vi "PressureCal.vi"(8 "Motion Settings In":T5={"No Motion?"=FALSE, "Motion System"=enum."No Motion Card", "Motion Bd ID"=1, "Motion Profile"="SMAC1", "# Axis"=1, "Reverse Z axis?"=TRUE, "SMAC Axis"=0, "scan pair"=enum."y-(x) scan", "RT fps"=6.0, "Steps per mm"=[1000, 1000, 1000, 1000], "Motor Parameters"={"velocity ct/s"=[10000.0, 10000.0, 10000.0, 50000.0], "accel ct/s^2"=[50000.0, 50000.0, 50000.0, 200000.0]}, "One Way Scan"=FALSE, "Reverse One Way Scan"=FALSE, "Global Position (mm)"=[], "Plane"=0, "Distance between\nscan lines (um)"=0.0, "Distance between\nscan planes (um)"=0.0, "number of scan planes"=1, "Total steps in line"=0, "Xtra plane\ndistance  (um)"=100, "Xtra planes "=1, "Add Axis"=FALSE, "overshoot cts"=200, "BKPT Shift"=0, "Scan Start Time (ms)"=0, "ESP VISA"="GPIB::1::INSTR", "3rd Axis"=1, "GL Ref Out"=refnum, "Galil Address"=""} {"3rd Axis" items=["x", "y", "z", "w"]; "Xtra planes" min=1; "Xtra plane\ndistance  (um)" min=0; "Distance between\nscan planes (um)" format="%.2f"; "Distance between\nscan lines (um)" format="%.2f"; "SMAC Axis" items=["None"=0, "Axis 1"=1, "Axis 2"=2, "Axis 3"=3, "Axis 4"=4, "Axis 5"=5, "Axis 6"=6, "Axis 7"=7, "Axis 8"=8, "Vector Space 1"=17, "Vector Space 2"=18, "Vector Space 3"=19, "Vector Space 4"=20]; "Motion Bd ID" min=1 max=32 step=1}, 9 "Burst Select":bool=TRUE, 10 "FG Source":u16(ring)=1 items=["Agilent"=2, "Tabor"=7, ""=0], 11 "Digitizer Settings":T1={"Digitizer delay (us) "=0.0, "rf points per line"=2048, "lines per plane"=128, "Samp Rate (Hz)"=100000000.0, "Additional dig delay (us)"=0.0, "Voltage Scale"=0.4, "Pre-Looks"=0, "Offset delay (us)"=0.0, "bits A/D"=8, "Avg Num"=1, "DigTimeOut"=5.0, "Rel Dig Delay"=0.0, "Dig Ch"=0, "LeCroyCluster"={"LeCroy Channels"=[TRUE, FALSE, FALSE, FALSE], "LC read pt offset"=0.0, "Sweep Avg"=FALSE}, "Main Digitizer"=enum."NI Digitizer", "Dig Config"=enum."Single channel", "Digitizer ID Cluster"={"Acqiris/Alazar/SP ID"=[], "NI Instr Handles"=[], "LeCroy VISA"="", "GaGe Handle"={"Handle"=0, "Sample size"=0, "Resolution"=0, "Offset"=0, "Channels"=0, "Boards"=0}, "ATS Ref"="ATS9350", "Acqiris Address"=["PCI::INSTR0"], "ADQRef"=refnum, "adq_cu_ptr"=refnum}, "Trigger Settings"={"Trig Source"=1, "Trig Coupling"=0, "Trig Slope"=0, "Level (mV)"=1500.0}, "Bulk Acq"=FALSE, "Bulk Start Indexes"=[], "Data Ref RF"=refnum, "NI ID/Channel"=[], "Total Dig CH"=5, "Xtra Ann Trig delay (us)"=10.0, "Fix Z Delay?"=FALSE, "One Way Transmission?"=FALSE, "Data Ref Log"=refnum} {"Trigger Settings"."Trig Slope" items=["Positive", "Negative"]; "Trigger Settings"."Level (mV)" format="%.2f"; "Trigger Settings"."Trig Coupling" items=["DC 1 MOhm", "AC 1 MOhm", "DC 50 Ohm", "AC 50 Ohm"]; "Trigger Settings"."Trig Source" items=["Chan 1", "External"]; "Rel Dig Delay" format="%.2f"; "DigTimeOut" format="%.2f"; "Avg Num" min=1; "Offset delay (us)" format="%.2f"; "Additional dig delay (us)" format="%.2f"; "Digitizer delay (us)" format="%.2f"}) -> (0 "Motion Settings Out":T5={"No Motion?"=FALSE, "Motion System"=enum."No Motion Card", "Motion Bd ID"=1, "Motion Profile"="SMAC1", "# Axis"=1, "Reverse Z axis?"=TRUE, "SMAC Axis"=0, "scan pair"=enum."y-(x) scan", "RT fps"=6.0, "Steps per mm"=[1000, 1000, 1000, 1000], "Motor Parameters"={"velocity ct/s"=[10000.0, 10000.0, 10000.0, 50000.0], "accel ct/s^2"=[50000.0, 50000.0, 50000.0, 200000.0]}, "One Way Scan"=FALSE, "Reverse One Way Scan"=FALSE, "Global Position (mm)"=[], "Plane"=0, "Distance between\nscan lines (um)"=0.0, "Distance between\nscan planes (um)"=0.0, "number of scan planes"=1, "Total steps in line"=0, "Xtra plane\ndistance  (um)"=100, "Xtra planes "=1, "Add Axis"=FALSE, "overshoot cts"=200, "BKPT Shift"=0, "Scan Start Time (ms)"=0, "ESP VISA"="GPIB::1::INSTR", "3rd Axis"=1, "GL Ref Out"=refnum, "Galil Address"=""} {"3rd Axis" items=["x", "y", "z", "w"]; "Xtra planes" min=1; "Xtra plane\ndistance  (um)" min=0; "Distance between\nscan planes (um)" format="%.2f"; "Distance between\nscan lines (um)" format="%.2f"; "SMAC Axis" items=["None"=0, "Axis 1"=1, "Axis 2"=2, "Axis 3"=3, "Axis 4"=4, "Axis 5"=5, "Axis 6"=6, "Axis 7"=7, "Axis 8"=8, "Vector Space 1"=17, "Vector Space 2"=18, "Vector Space 3"=19, "Vector Space 4"=20]; "Motion Bd ID" min=1 max=32 step=1}, 3 "Digitizer Settings Out":T1={"Digitizer delay (us) "=0.0, "rf points per line"=2048, "lines per plane"=128, "Samp Rate (Hz)"=100000000.0, "Additional dig delay (us)"=0.0, "Voltage Scale"=0.4, "Pre-Looks"=0, "Offset delay (us)"=0.0, "bits A/D"=8, "Avg Num"=1, "DigTimeOut"=5.0, "Rel Dig Delay"=0.0, "Dig Ch"=0, "LeCroyCluster"={"LeCroy Channels"=[TRUE, FALSE, FALSE, FALSE], "LC read pt offset"=0.0, "Sweep Avg"=FALSE}, "Main Digitizer"=enum."NI Digitizer", "Dig Config"=enum."Single channel", "Digitizer ID Cluster"={"Acqiris/Alazar/SP ID"=[], "NI Instr Handles"=[], "LeCroy VISA"="", "GaGe Handle"={"Handle"=0, "Sample size"=0, "Resolution"=0, "Offset"=0, "Channels"=0, "Boards"=0}, "ATS Ref"="ATS9350", "Acqiris Address"=["PCI::INSTR0"], "ADQRef"=refnum, "adq_cu_ptr"=refnum}, "Trigger Settings"={"Trig Source"=1, "Trig Coupling"=0, "Trig Slope"=0, "Level (mV)"=1500.0}, "Bulk Acq"=FALSE, "Bulk Start Indexes"=[], "Data Ref RF"=refnum, "NI ID/Channel"=[], "Total Dig CH"=5, "Xtra Ann Trig delay (us)"=10.0, "Fix Z Delay?"=FALSE, "One Way Transmission?"=FALSE, "Data Ref Log"=refnum} {"Trigger Settings"."Trig Slope" items=["Positive", "Negative"]; "Trigger Settings"."Level (mV)" format="%.2f"; "Trigger Settings"."Trig Coupling" items=["DC 1 MOhm", "AC 1 MOhm", "DC 50 Ohm", "AC 50 Ohm"]; "Trigger Settings"."Trig Source" items=["Chan 1", "External"]; "Rel Dig Delay" format="%.2f"; "DigTimeOut" format="%.2f"; "Avg Num" min=1; "Offset delay (us)" format="%.2f"; "Additional dig delay (us)" format="%.2f"; "Digitizer delay (us)" format="%.2f"})   [LabVIEW 2022 SP3]
uses:
  -CalTransducer/HydrophoneSettings.ctl
  -CalTransducer/Hydros.ctl
  ScanningControl/Digitizers/-DigitizerRoutines/DigitizerSettings.ctl
  ScanningControl/Digitizers/-DigitizerRoutines/Digitizer.ctl
  ScanningControl/Digitizers/-DigitizerRoutines/DigConfig.ctl
  ScanningControl/Digitizers/-DigitizerRoutines/DigitizerID.ctl
  C:/Windows/System32/ADQAPI_dotNet_helper.dll
  ScanningControl/Motion Controllers/NI_controller/-NI_MotionRoutines/MotionParameters.ctl
  ScanningControl/Motion Controllers/NI_controller/-NI_MotionRoutines/MotionSys.ctl
  ScanningControl/Motion Controllers/-MotionRoutines/ScanAxis.ctl
  ScanningControl/Motion Controllers/-MotionRoutines/3rdAxis.ctl
  ScanningControl/-ScanSystem/Controls/ScanType2.ctl
  <vilib>/DAQmx/write.llb/DAQmx Write (Digital 1D Bool NChan 1Samp 1Line).vi
  <vilib>/Analysis/5stat.llb/RMS (DBL).vi
  <vilib>/Analysis/baseanly.llb/Mean (DBL).vi
  <vilib>/DAQmx/miscellaneous.llb/DAQmx Fill In Error Info.vi
  <instrlib>/niScope/Acquire/Fetch/niScope Fetch.vi
  <vilib>/Utility/file.llb/Write Delimited Spreadsheet (DBL).vi
  <instrlib>/Acqiris Dx/Acqiris Dx.lvlib
  <vilib>/Analysis/NI_AALPro.lvlib
  <vilib>/Analysis/NI_AALBase.lvlib
panel:
  in  "Invert PAL voltage":bool=TRUE
  out "f (MHz)":dbl
  in  "Freq Step to View":u8
  in  "V probe":u16(ring)=1 items=["1x"=1, "10x"=10, "100x"=100]
  in  "Start freq (MHz)":dbl=1.0 format="%.2f"
  in  "Freq Steps":u32=1
  in  "Average":i32=1
  in  "Freq Step (MHz":dbl=2.0 format="%.2f"
  in  "Cal Tran":bool
  in  "Set up Digi":bool
  in  "ExitSendCmd":bool
  in  "Save Cal Data":bool
  in  "Save RF array?":bool
  in  "Pressure Cal Parameters":T9={"Center Freq (MHz)"=40.0, "PRF (kHz)"=1.0, "Pulse window (us)"=0.5, "Hydrophone"=enum."DEAD PAL # 1403", "booster amp?"=TRUE} {"Pulse window (us)" format="%.2f"; "PRF (kHz)" format="%.2f"; "Center Freq (MHz)" format="%.2f"}
  in  "Voltage Step (mVpp)":dbl=10.0 format="%.2f"
  in  "Voltage Steps":i32=20
  in  "Start voltage (mVpp)":dbl=50.0 format="%.3f"
  out "RMS dB ratio":cluster{"V Steps":dbl[], "RMS Ratio":dbl[]}(graph)
  out "current f (MHz)":dbl
  out "Voltage + pk and -pk":dbl[][](graph)
  out "Raw RF":dbl[][](array[numeric])
  out "Cal Array":dbl[][](array[numeric])
  out "Mpa/V":dbl format="%.2f"
  out "Voltage at Transducer":cluster{dbl[], dbl[]}(graph)
  out "Hydrophone":cluster{"V Steps":dbl[], dbl[]}[](graph)
  out "slope":dbl format="%.2f"
  out "intercept":dbl format="%.2f"
  out "mse":dbl format="%.2f"
  out "current Vpp":dbl
  # "***Voltages are inverted for PAL 40 um hydrophones***"
  # ")"
  # "Fit Params for hydrophone"
  # "FG drive\nvoltage matching (Vpp)\nvolt hydrop V\nPressure  neg MPa"
  # "1-D and 2-D B scan settings"
  # "1-D and 2-D B scan settings"
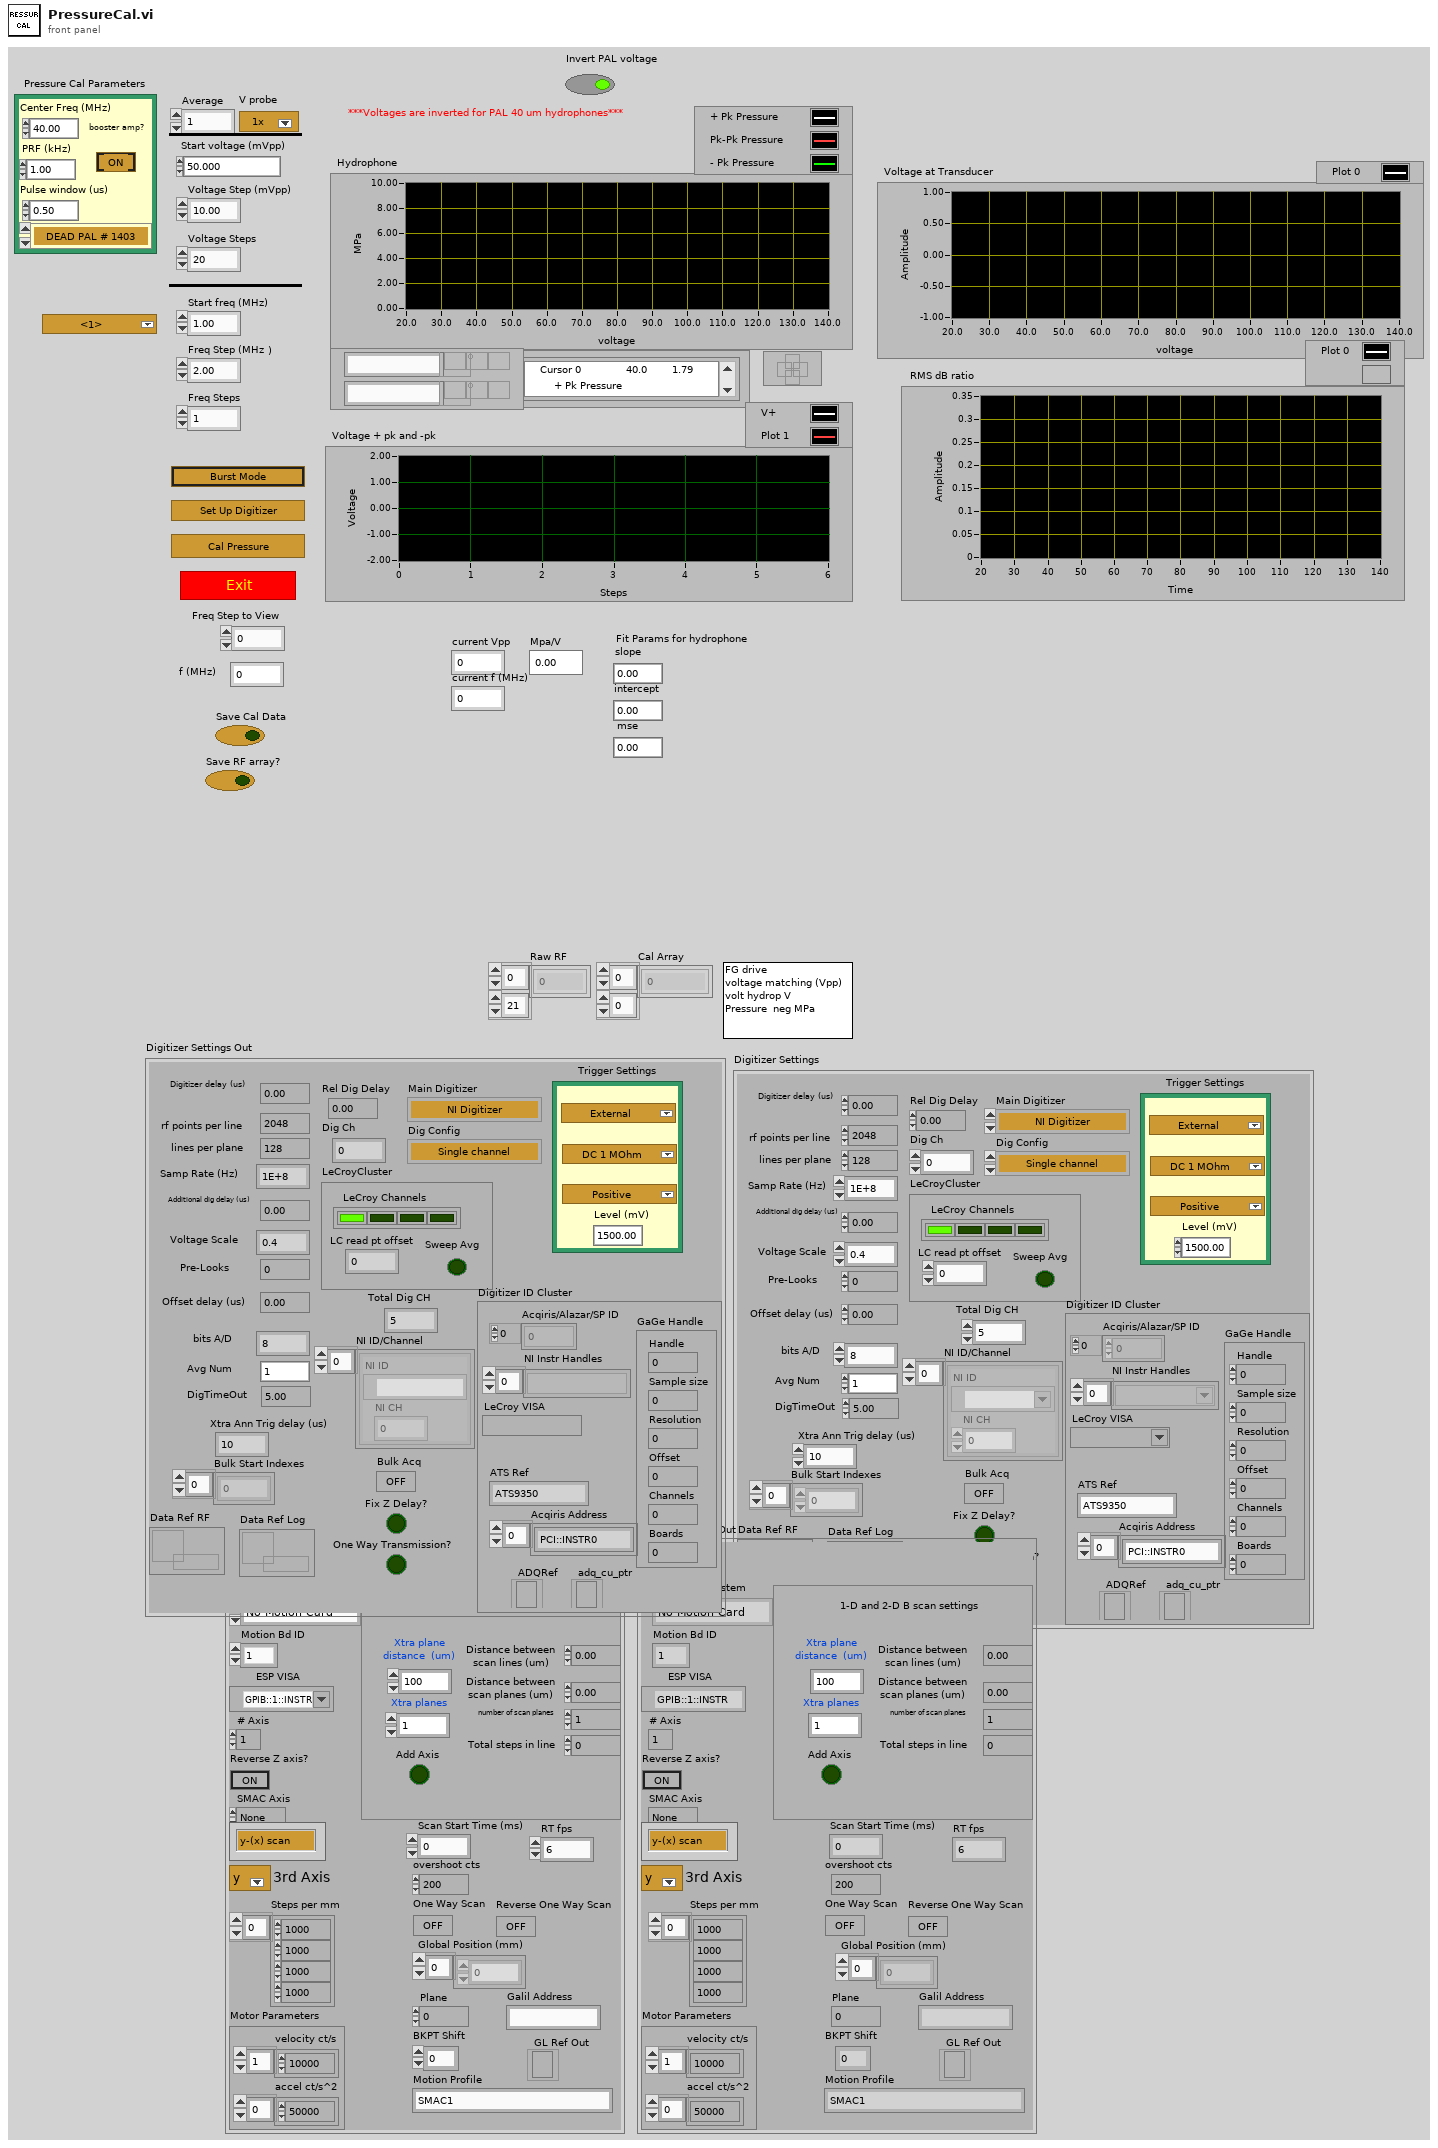
[diagram p1: front panel]
types:
  T1 = typedef "DigitizerSettings.ctl" = cluster{"Digitizer delay (us) ":dbl, "rf points per line":i32, "lines per plane":i32, "Samp Rate (Hz)":dbl, "Additional dig delay (us)":dbl, "Voltage Scale":dbl, "Pre-Looks":i32, "Offset delay (us)":dbl, "bits A/D":i8, "Avg Num":i32, "DigTimeOut":sgl, "Rel Dig Delay":sgl, "Dig Ch":i32, "LeCroyCluster":cluster{"LeCroy Channels":bool[], "LC read pt offset":dbl, "Sweep Avg":bool}, "Main Digitizer":T2, "Dig Config":T3, "Digitizer ID Cluster":T4, "Trigger Settings":cluster{"Trig Source":u16, "Trig Coupling":u16, "Trig Slope":u16, "Level (mV)":dbl}, "Bulk Acq":bool, "Bulk Start Indexes":i32[], "Data Ref RF":refnum<data-value>, "NI ID/Channel":cluster{"NI ID":refnum<k15>, "NI CH":i32}[], "Total Dig CH":i32, "Xtra Ann Trig delay (us)":dbl, "Fix Z Delay?":bool, "One Way Transmission?":bool, "Data Ref Log":refnum<data-value>}
  T2 = typedef "Digitizer.ctl" = enum16{"Acqiris Digitizer", "NI Digitizer", "LeCroy", "GaGe", "AlazarTech", "No Digitizer", "Teledyne"}
  T3 = typedef "DigConfig.ctl" = enum16{"Single channel", "2 Chans w/ 2 Acqiris", "2 Chans w/ 1 Acqiris", "5-CH Pulser New", "5-CH pulser w/ ann array", "5-pass style ann array", "Empty"}
  T4 = typedef "DigitizerID.ctl" = cluster{"Acqiris/Alazar/SP ID":u32[], "NI Instr Handles":refnum<k15>[], "LeCroy VISA":refnum<visa-resource-name>, "GaGe Handle":cluster{"Handle":u32, "Sample size":u32, "Resolution":i32, "Offset":i32, "Channels":u32, "Boards":u32}, "ATS Ref":string, "Acqiris Address":string[], "ADQRef":refnum<k24>, "adq_cu_ptr":refnum<k24>}
  T5 = typedef "MotionParameters.ctl" = cluster{"No Motion?":bool, "Motion System":T6, "Motion Bd ID":u8, "Motion Profile":string, "# Axis":i8, "Reverse Z axis?":bool, "SMAC Axis":u16, "scan pair":T7, "RT fps":sgl, "Steps per mm":i32[], "Motor Parameters":cluster{"velocity ct/s":dbl[], "accel ct/s^2":dbl[]}, "One Way Scan":bool, "Reverse One Way Scan":bool, "Global Position (mm)":dbl[], "Plane":i32, "Distance between\nscan lines (um)":sgl, "Distance between\nscan planes (um)":sgl, "number of scan planes":i32, "Total steps in line":i32, "Xtra plane\ndistance  (um)":i32, "Xtra planes ":i32, "Add Axis":bool, "overshoot cts":i32, "BKPT Shift":i32, "Scan Start Time (ms)":u32, "ESP VISA":refnum<visa-resource-name>, "3rd Axis":T8, "GL Ref Out":refnum<k7>, "Galil Address":string}
  T6 = typedef "MotionSys.ctl" = enum16{"MM3000", "NI 735x", "Newport ESP", "No Motion Card", "Galil"}
  T7 = typedef "ScanAxis.ctl" = enum16{"y-(x) scan", "x-(y) scan", "z-(x) scan", "z-(y) scan", "y-(z) scan", "x-(z) scan", "w-(x) scan", "w-(y) scan", "w-(z) scan", "x-(w) scan", "y-(w) scan", "z-(w) scan"}
  T8 = typedef "3rdAxis.ctl" = u16
  T9 = typedef "HydrophoneSettings.ctl" = cluster{"Center Freq (MHz)":dbl, "PRF (kHz)":dbl, "Pulse window (us)":dbl, "Hydrophone":T10, "booster amp?":bool}
  T10 = typedef "Hydros.ctl" = enum16{"PAL #1048", "PAL #525", "PAL #430a", "PAL #192", "DEAD PAL # 1403", "LOST UHI Onda", "DEAD PAL #1818", "PAL #1974", "DEAD #2266 w/booster", "PAL #2524 w/booster", "PAL FP21-20T", "PAL FP160-13  ", "PAL FP141-20", "PAL FP158-08T"}
  T11 = cluster{"+ pk Ch1":dbl[], "Pk-Pk Ch1":dbl[], "-Pk Ch1":dbl[], "V Steps":dbl[], "WaveForms Ch1":dbl[][], "RMS Ch1":dbl[], "+  pk Ch2":dbl[], "RMS Ch2":dbl[], "RMS Ratio":dbl[], "freq":dbl}
  T12 = typedef "ScanType2.ctl" = enum16{"Therapy With Scan", "M scan", "M Scan With Therapy Burst", "1-D B Scan", "1-D B Scan With Therapy Burst", "2-D B Scan", "2-D B Scan With Therapy Burst", "Rotational Scan", "1-D B-Scan PRF", "2-D B-Scan PRF", "Real-Time Scan", "Contrast Agents", "1-D w/ Real-Time Set Up", "Dual Transducer", "Acoustic Microscopy", "Hydrophone Scanning"}
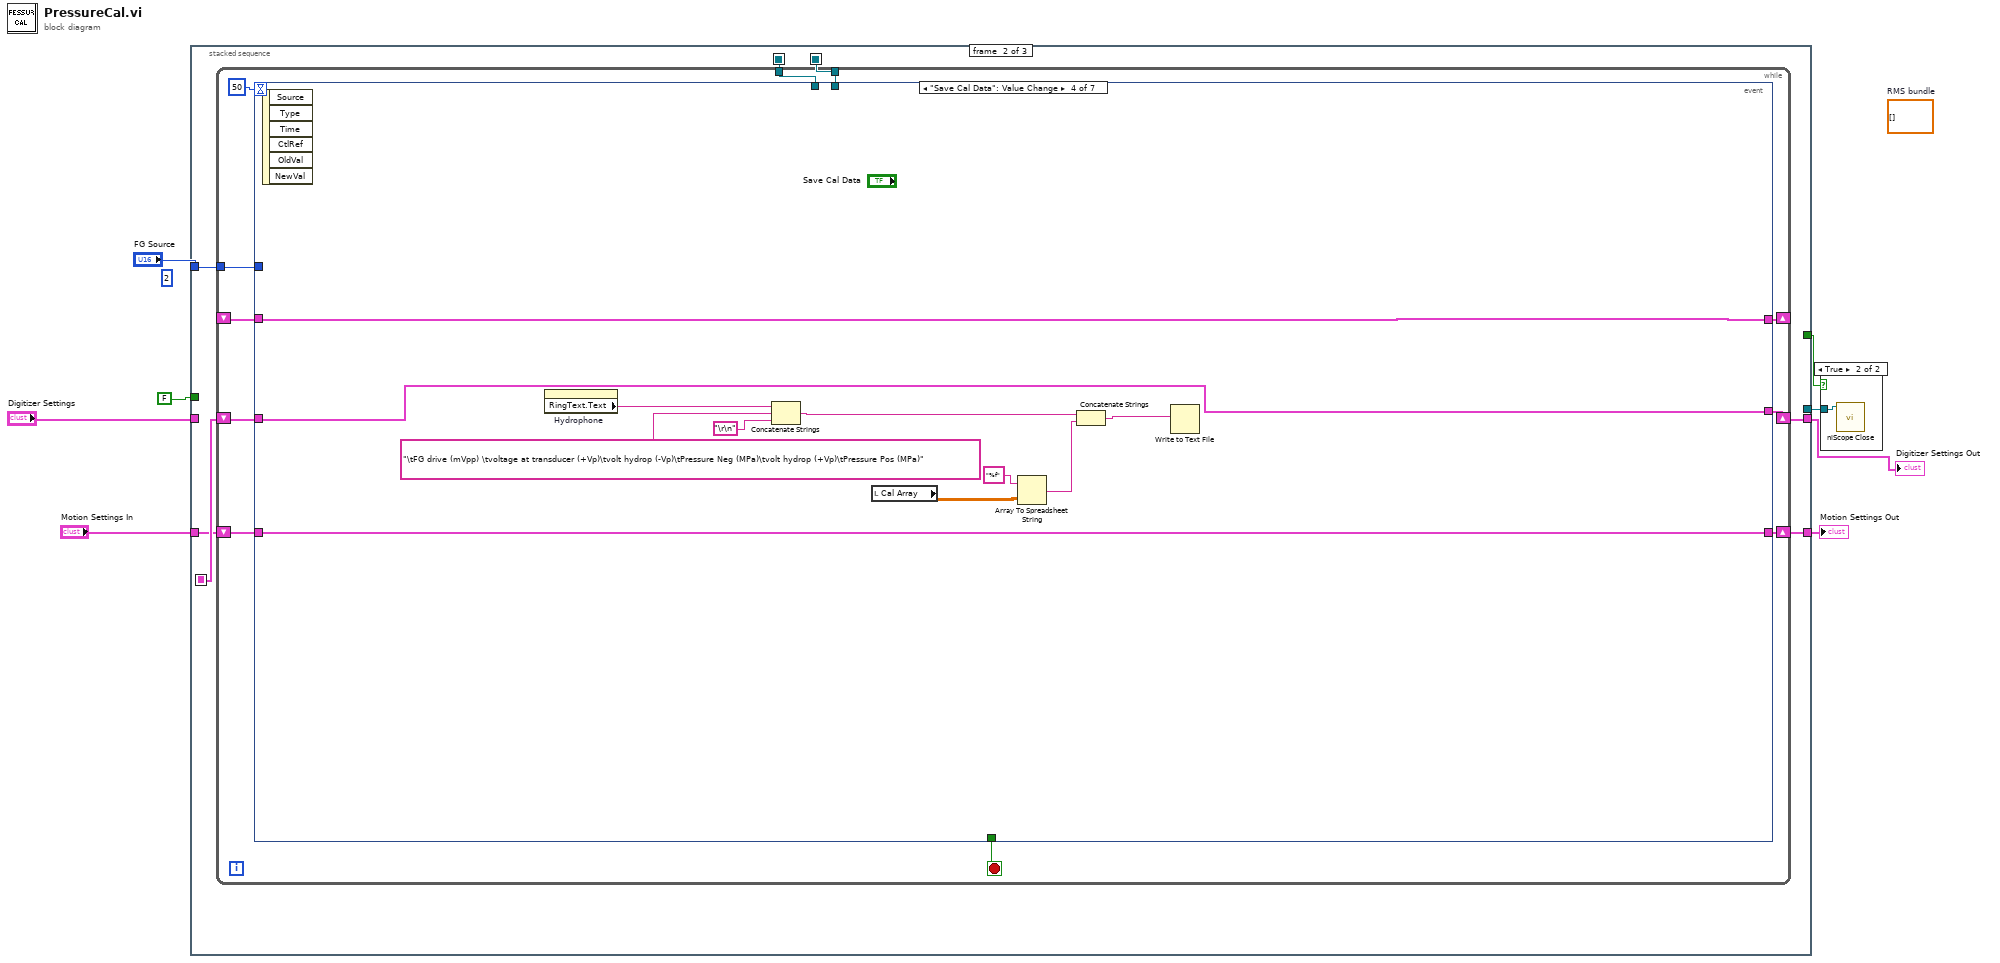
[diagram p0: block diagram]
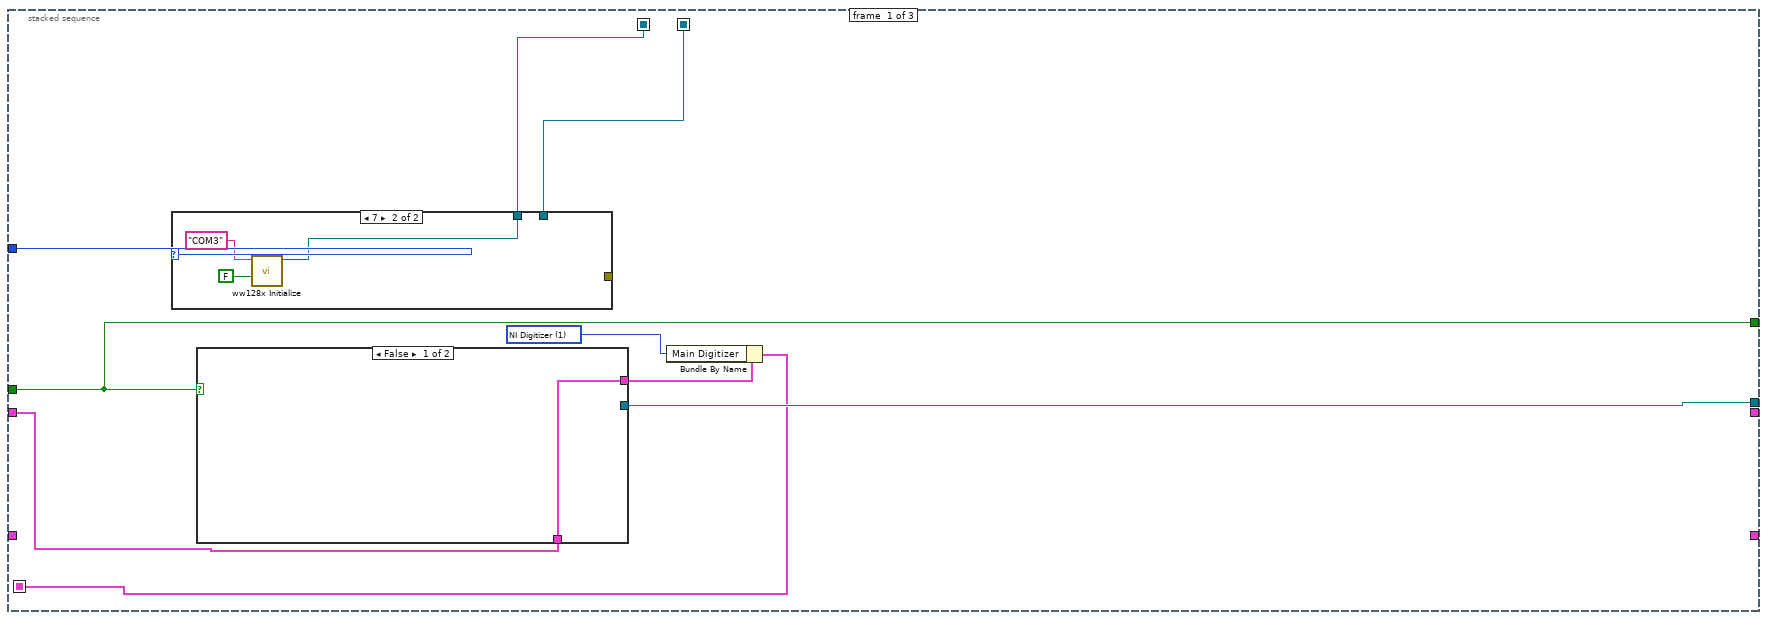
[diagram p3: hidden frame]
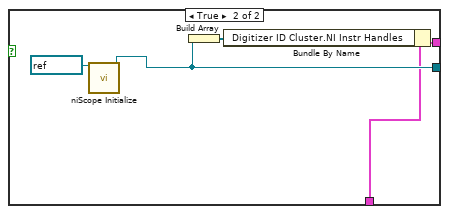
[diagram p4: hidden frame]
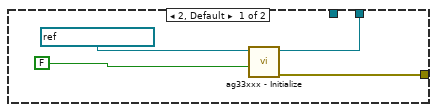
[diagram p5: hidden frame]
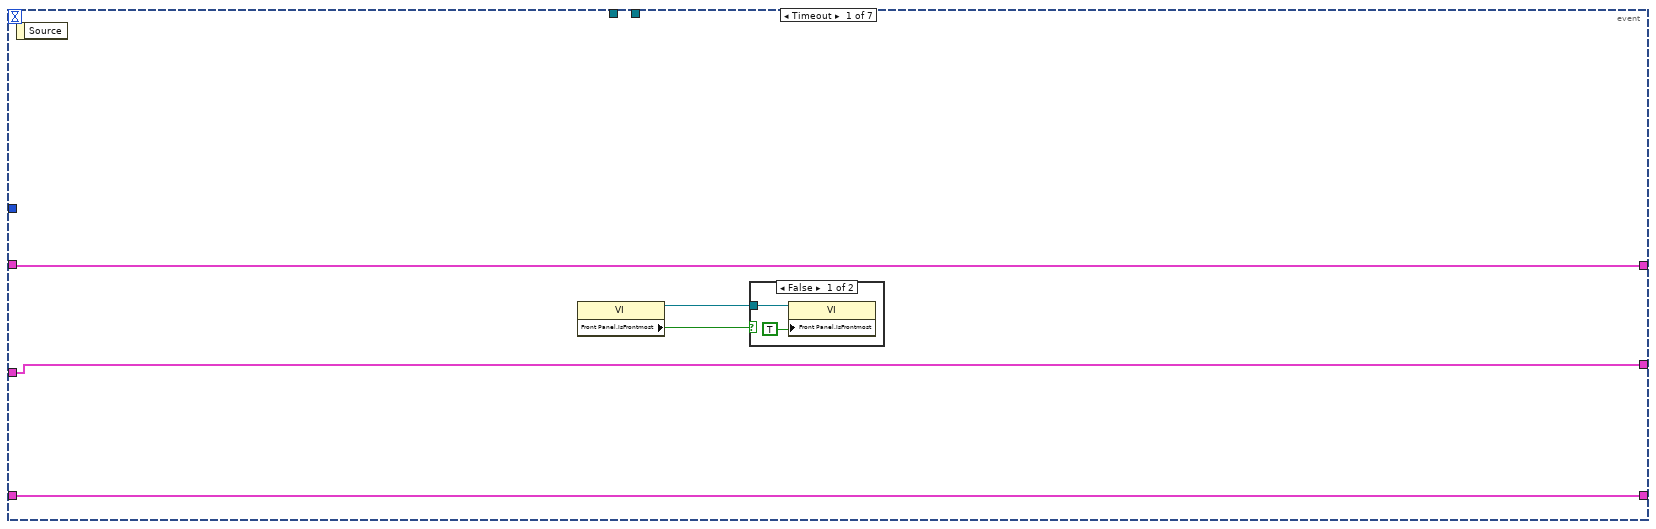
[diagram p6: hidden frame]
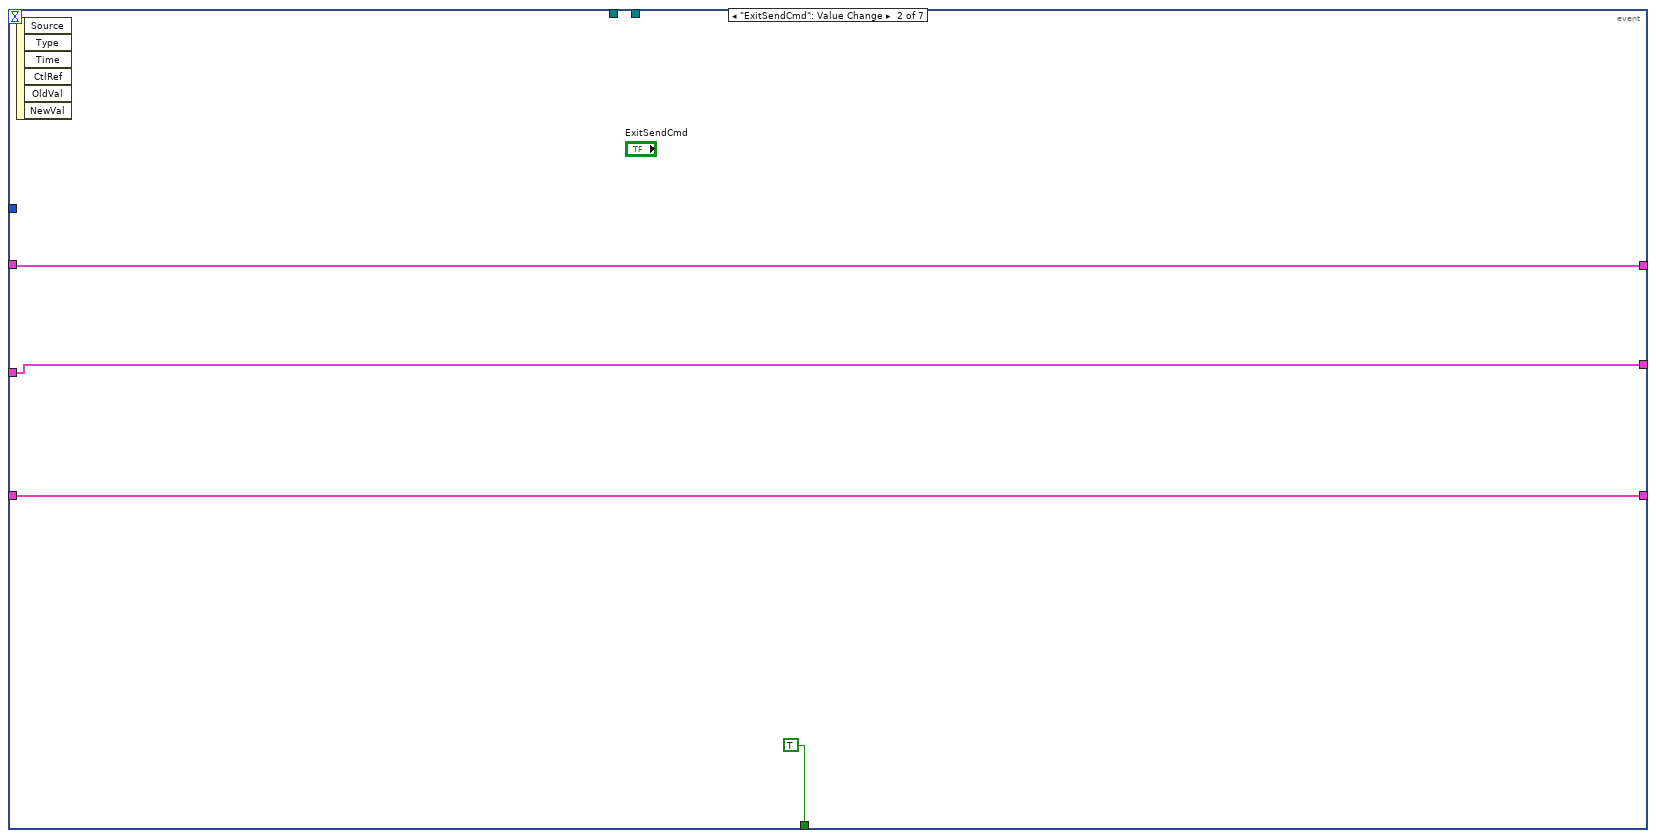
[diagram p8: hidden frame]
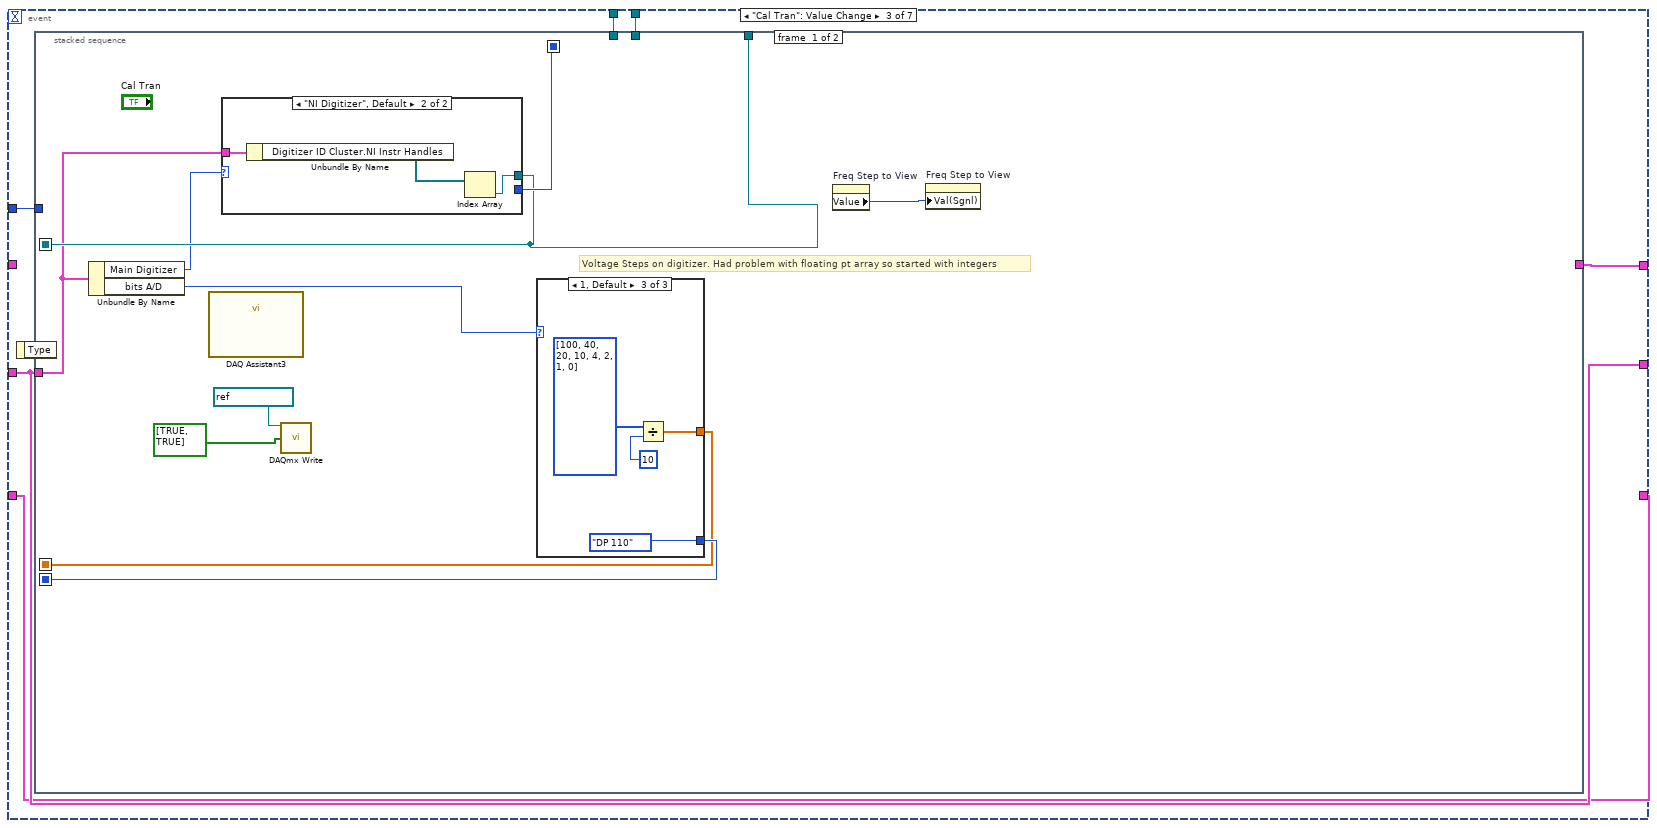
[diagram p9: hidden frame]
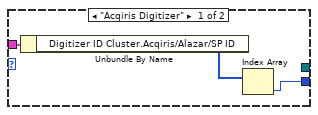
[diagram p10: hidden frame]
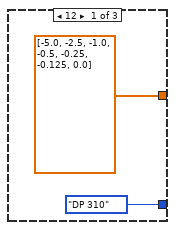
[diagram p11: hidden frame]
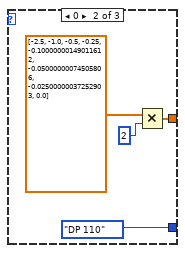
[diagram p12: hidden frame]
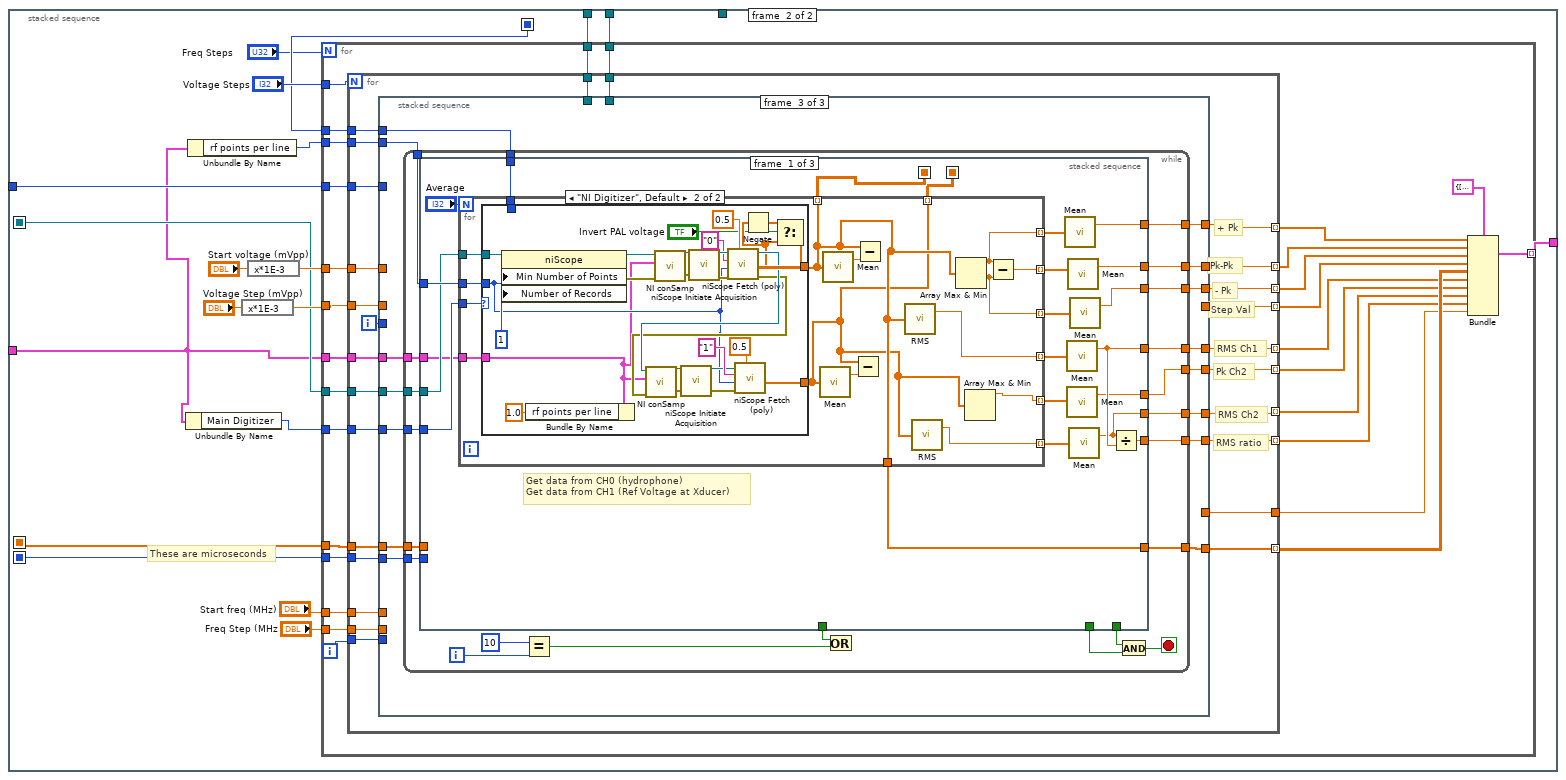
[diagram p13: hidden frame]
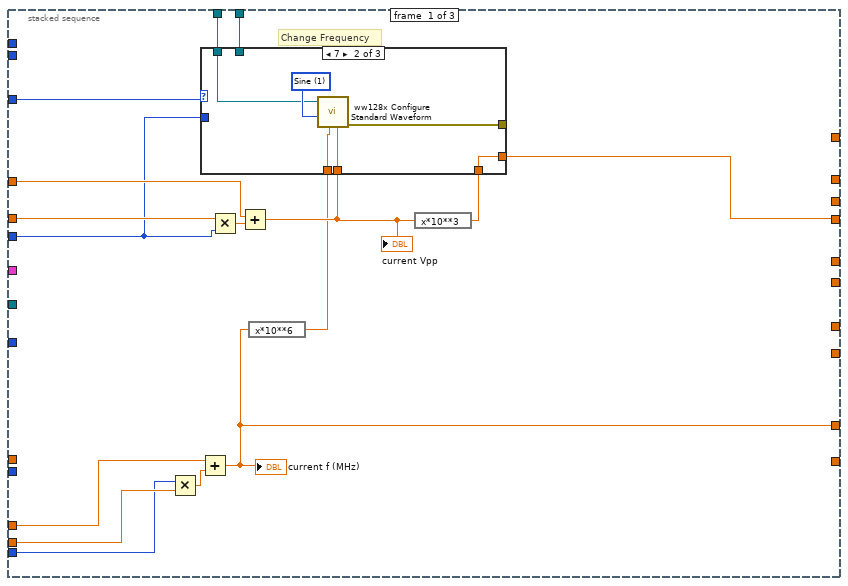
[diagram p14: hidden frame]
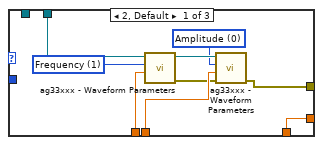
[diagram p15: hidden frame]
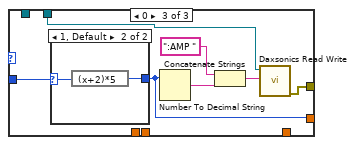
[diagram p16: hidden frame]
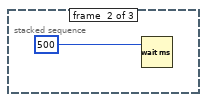
[diagram p18: hidden frame]
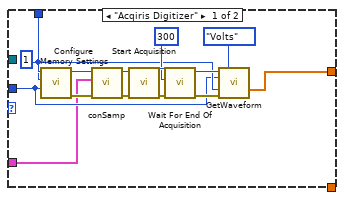
[diagram p19: hidden frame]
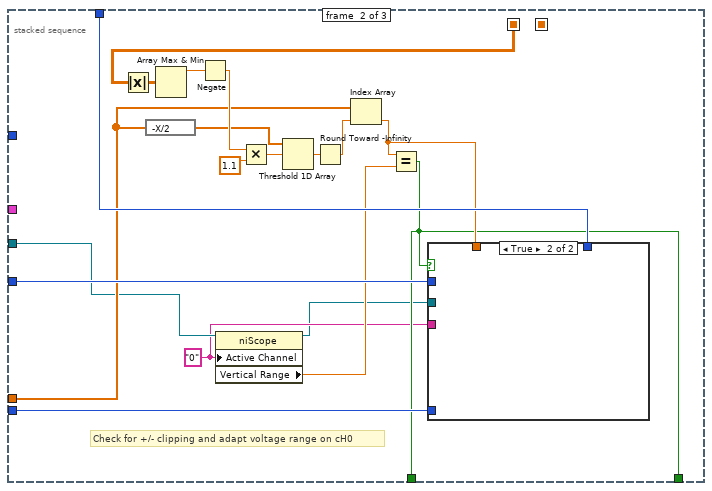
[diagram p20: hidden frame]
diagram:
  (unwired) 2
  (unwired) dbl[][] []  # RMS bundle
  n1 = stacked-sequence {
    seq-local: [w15 _ _] -> [_ w36 w459]
    seq-local: [w16 _ _] -> [_ w35 w458]
    seq-local: [w10 _ _] -> [_ w34 _]
    tunnel: "FG Source" -> [w17 w37 w460]
    tunnel: [w14 _ _] -> w8
    tunnel: FALSE -> [w13 _ w457]
    tunnel: [w13 _ _] -> w6
    tunnel: "Digitizer Settings" -> [w12 _ _]
    tunnel: "Motion Settings In" -> [_ w33 _]
    tunnel: [_ w32 _] -> w2
    tunnel: [_ w31 _] -> w1
    frame #0 {
      w9 = u16 1 items=["Acqiris Digitzer", "NI Digitizer"] ("Main Digitizer")
      n2 = case shown="7" w17 {
        tunnel: [w26 _] -> w16
        tunnel: [_ w28] -> w15
        tunnel: [w24 _] -> _
        frame 2, Default {
          n3 = call <instrlib>:"ag33xxx - Initialize.vi"("Reset (T: Reset)"=FALSE, "Instrument Resource Name"=refnum<visa-resource-name> "GPIB0::10::INSTR") -> ("error out"=w24:errorcluster, "dup VISA session"=w26:refnum<visa-resource-name>)  [unwired: 8 in]
        }
        frame 7 {
          n4 = call <instrlib>:"ww128x Initialize.vi"("reset device (Yes)"=FALSE ("reset device"), "resource name"="COM3") -> ("instrument handle out"=w28:refnum<k15>)  [unwired: 2 in, 7 out]
        }
      }
      n5 = case shown="False" w13 {
        tunnel: [_ w22] -> w14
        tunnel: w12 -> [w18 w20]
        tunnel: [w18 w19] -> w11
        frame False {
        }
        frame True {
          n6 = call <instrlib>:"niScope Initialize.vi"("resource name"=refnum<k15> "Dig1") -> ("instrument handle"=w22:refnum<k15>)  [unwired: 3 in, 11 out]
          n7 = Build Array(w22) -> (w21:refnum<k15>[])
          n8 = Bundle By Name(cluster=w20, "Digitizer ID Cluster.NI Instr Handles"=w21) -> (w19:T1)
        }
      }
      n9 = Bundle By Name(cluster=w11, "Main Digitizer"=w9) -> (w10:T1)
    }
    frame #1 {
      n10 = while {
        tunnel: w37 -> [w46]
        tunnel: w36 -> [w45]
        tunnel: w35 -> [w44]
        shift-right: [w43] -> _
        shift-left: _ -> [w42]
        shift-right: [w39] -> w32
        shift-left: w33 -> [w40]
        shift-right: [w38] -> w31
        shift-left: w34 -> [w41]
        stop <- w48 stop-if-true
        n11 = event shown="[3] \"Save Cal Data\": Value Change" {
          selector: _ -> [_ _ _ _ _ _ _]
          dyn-events: _ -> [_ _ _ _ _ _ _]
          timeout: 50 -> [_ _ _ _ _ _ _]
          tunnel: [_ TRUE _ _ _ _ _] -> w48
          tunnel: w46 -> [_ _ w65 _ _ _ _]
          tunnel: w45 -> [_ _ w64 _ _ _ _]
          tunnel: w44 -> [_ _ w63 _ _ _ _]
          tunnel: [w51 w58 w62 w374 w377 w385 w400] -> w43
          tunnel: w42 -> [w51 w58 _ w374 w377 w385 w400]
          tunnel: w41 -> [w49 w56 w61 w364 w375 w384 w388]
          tunnel: w40 -> [w50 w57 w60 w365 w376 w383 w389]
          tunnel: [w50 w57 w60 w365 w376 w382 w389] -> w39
          tunnel: [w49 w56 w61 w364 w375 w381 w388] -> w38
          event Timeout {
            n12 = event-data() -> ()  [unwired: 2 out]
            n13 = property class="VI"() -> (reference out=w53:refnum<vi>, "Front Panel.IsFrontmost"=w52:bool)  [unwired: 2 in, 1 out]
            n14 = case shown="False" w52 {
              tunnel: w53 -> [w55 _]
              frame False {
                n15 = property class="VI"(reference=w55, "Front Panel.IsFrontmost"=TRUE) -> ()  [unwired: 1 in, 2 out]
              }
              frame True {
              }
            }
          }
          event "ExitSendCmd": Value Change {
            n16 = event-data() -> ()  [unwired: 7 out]
          }
          event "Cal Tran": Value Change {
            n17 = event-data() -> ()  [unwired: 2 out]
            n18 = stacked-sequence {
              seq-local: [w74 _] -> [_ w108]
              seq-local: [w75 _] -> [_ w109]
              seq-local: [w73 _] -> [_ w103]
              seq-local: [w69 _] -> [_ w102]
              tunnel: w65 -> [_ w101]
              tunnel: w64 -> [_ w100]
              tunnel: w63 -> [_ w99]
              tunnel: [_ w95] -> w62
              tunnel: [w69 _] -> _
              tunnel: w61 -> [w68 w93]
              frame #0 {
                # "Voltage Steps on digitizer. Had problem with floating pt array so started with integers"
                n19 = Unbundle By Name(w68) -> ("Main Digitizer"=w67:T2, "bits A/D"=w66:i8)
                n20 = call "DAQ Assistant3"() -> ()  [unwired: 17 in, 3 out]
                n21 = case shown="\"NI Digitizer\", Default" w67 {
                  tunnel: [w77 _] -> w73
                  tunnel: [_ w80] -> w69
                  tunnel: w68 -> [w76 w79]
                  frame "Acqiris Digitizer" {
                    n22 = Unbundle By Name(w76) -> ("Digitizer ID Cluster.Acqiris/Alazar/SP ID"=w78:u32[])
                    n23 = Index Array(array=w78) -> (element=w77:u32)  [unwired: 1 in]
                  }
                  frame "NI Digitizer", Default {
                    n24 = Unbundle By Name(w79) -> ("Digitizer ID Cluster.NI Instr Handles"=w81:refnum<k15>[])
                    n25 = Index Array(array=w81) -> (element=w80:refnum<k15>)  [unwired: 1 in]
                  }
                }
                n26 = call-poly <vilib>:"DAQmx Write.vi"("task/channels in"=refnum<k21> "DIO-L2 L3", "data"=bool[] [TRUE, TRUE]) -> ()  [unwired: 11 in, 3 out]
                n27 = case shown="1, Default" w66 {
                  tunnel: [sgl[] [-5.0, -2.5, -1.0, -0.5, -0.25, -0.125, 0.0] w84 w89] -> w74
                  tunnel: [enum16{"DP 110", "DP 310"}."DP 310" ("Card Type") enum16{"DP 110", "DP 310"}."DP 110" ("Card Type") enum16{"DP 110", "DP 310"}."DP 110" ("Card Type")] -> w75
                  frame 12 {
                  }
                  frame 0 {
                    n28 = Multiply(x=sgl[] [-2.5, -1.0, -0.5, -0.25, -0.1, -0.05, -0.025, 0.0], y=2) -> (x*y=w84:sgl[])
                  }
                  frame 1, Default {
                    n29 = Divide(x=i32[] [100, 40, 20, 10, 4, 2, 1, 0] ("32bit integer"), y=10) -> (x/y=w89:dbl[])
                  }
                }
                n30 = property on="Freq Step to View" class="DigNum (strict)"() -> ("Value"=w70:u8)  [unwired: 2 in, 2 out]
                n31 = property on="Freq Step to View" class="DigNum (strict)"("Val(Sgnl)"=w70) -> ()  [unwired: 2 in, 2 out]
              }
              frame #1 {
                # "These are microseconds"
                n32 = Unbundle By Name(w93) -> ("Main Digitizer"=w92:T2)
                n33 = Unbundle By Name(w93) -> ("rf points per line"=w94:i32)
                n34 = expression code="x*1E-3"("Voltage Step (mVpp)") -> (w106:dbl)
                n35 = expression code="x*1E-3"("Start voltage (mVpp)") -> (w104:dbl)
                n36 = for {
                  N: "Freq Steps" -> [_]
                  tunnel: "Voltage Steps" -> [w138]
                  tunnel: w94 -> [w137]
                  tunnel: w109 -> [w136]
                  tunnel: w108 -> [w135]
                  tunnel: w106 -> [w134]
                  tunnel: w104 -> [w133]
                  tunnel: w103 -> [w132]
                  tunnel: w92 -> [w128]
                  tunnel: [w127] -> w95 mode=indexing
                  tunnel: w102 -> [w126]
                  tunnel: w101 -> [w124]
                  tunnel: w100 -> [w123]
                  tunnel: w99 -> [w122]
                  tunnel: "Start freq (MHz)" -> [w120]
                  tunnel: "Freq Step (MHz" -> [w119]
                  tunnel: w93 -> [w111]
                  i -> [w121]
                  n37 = for {
                    N: w138 -> [_]
                    tunnel: w134 -> [w163]
                    tunnel: w133 -> [w162]
                    tunnel: [w161] -> w118 mode=indexing
                    tunnel: [w160] -> w125 mode=indexing
                    tunnel: w132 -> [w159]
                    tunnel: [w157] -> w131 mode=indexing
                    tunnel: w137 -> [w158]
                    tunnel: [w156] -> w130 mode=indexing
                    tunnel: [w155] -> w129 mode=indexing
                    tunnel: w124 -> [w154]
                    tunnel: w135 -> [w153]
                    tunnel: w136 -> [w152]
                    tunnel: w128 -> [w151]
                    tunnel: w126 -> [w150]
                    tunnel: [w149] -> w117 mode=indexing
                    tunnel: [w148] -> w116 mode=indexing
                    tunnel: [w147] -> w112 mode=indexing
                    tunnel: w123 -> [w146]
                    tunnel: w122 -> [w145]
                    tunnel: [w144] -> w114
                    tunnel: w121 -> [w143]
                    tunnel: w120 -> [w142]
                    tunnel: w119 -> [w141]
                    tunnel: [w140] -> w115 mode=indexing
                    tunnel: w111 -> [w139]
                    i -> [w164]
                    # "RMS Ch2"
                    # "RMS ratio"
                    # "Pk Ch2"
                    # "RMS Ch1"
                    # "Step Val"
                    # "- Pk"
                    # "Pk-Pk"
                    # "+ Pk"
                    n38 = stacked-sequence {
                      tunnel: w164 -> [w167 _ _]
                      tunnel: w163 -> [w180 _ _]
                      tunnel: w162 -> [w179 _ _]
                      tunnel: [_ _ w220] -> w161
                      tunnel: [w166 _ _] -> w160
                      tunnel: w159 -> [_ _ w221]
                      tunnel: w158 -> [_ _ w216]
                      tunnel: [_ _ w219] -> w157
                      tunnel: [_ _ w218] -> w156
                      tunnel: [_ _ w217] -> w155
                      tunnel: w154 -> [w177 _ _]
                      tunnel: w153 -> [_ _ w215]
                      tunnel: w152 -> [_ _ w214]
                      tunnel: w151 -> [_ _ w213]
                      tunnel: w150 -> [_ _ w212]
                      tunnel: [_ _ w211] -> w149
                      tunnel: [_ _ w210] -> w148
                      tunnel: [_ _ w209] -> w147
                      tunnel: w146 -> [w176 _ _]
                      tunnel: w145 -> [w175 _ _]
                      tunnel: [w173 _ _] -> w144
                      tunnel: w143 -> [w168 _ _]
                      tunnel: w142 -> [w170 _ _]
                      tunnel: w141 -> [w169 _ _]
                      tunnel: [_ _ w208] -> w140
                      tunnel: w139 -> [_ _ w207]
                      frame #0 {
                        # "Change Frequency"
                        n39 = Multiply(x=w168, y=w169) -> (x*y=w171:dbl)
                        n40 = Add(x=w170, y=w171) -> (x+y=w173:dbl)
                        "current f (MHz)" <- w173
                        n41 = Multiply(x=w180, y=w167) -> (x*y=w172:dbl)
                        n42 = Add(x=w179, y=w172) -> (x+y=w178:dbl)
                        "current Vpp" <- w178
                        n43 = expression code="x*10**6"(w173) -> (w174:dbl)
                        n44 = expression code="x*10**3"(w178) -> (w165:dbl)
                        n45 = case shown="7" w177 {
                          tunnel: w178 -> [w184 w195 _]
                          tunnel: w174 -> [w185 w193 _]
                          tunnel: w176 -> [_ w192 _]
                          tunnel: w175 -> [w189 _ w197]
                          tunnel: [w181 w191 w196] -> _
                          tunnel: w167 -> [_ _ w199]
                          tunnel: [w183 w190 w198] -> w166
                          tunnel: w165 -> [w183 w190 _]
                          frame 2, Default {
                            w186 = u16 0 items=["Amplitude", "Frequency", "Offset"] ("Parameter (0: Amplitude)")
                            w187 = u16 1 items=["Amplitude", "Frequency", "Offset"] ("Parameter (0: Amplitude)")
                            n46 = call <instrlib>:"ag33xxx - Waveform Parameters.vi"("Value (1.00)"=w185, "Parameter (0: Amplitude)"=w187, "VISA session"=w189) -> ("error out"=w182:errorcluster, "dup VISA session"=w188:refnum<visa-resource-name>)  [unwired: 7 in]
                            n47 = call <instrlib>:"ag33xxx - Waveform Parameters.vi"("error in (no error)"=w182, "Value (1.00)"=w184, "Parameter (0: Amplitude)"=w186, "VISA session"=w188) -> ("error out"=w181:errorcluster)  [unwired: 6 in, 1 out]
                          }
                          frame 7 {
                            w194 = 1 items=["Sine"=1, "Square"=2, "Triangle"=3, "Ramp Up"=4, "Ramp Down"=5, "DC"=6, "Ramp"=1001, "Pulse"=1005, "Sync"=1002, "Gaussian"=1003, "Exponential"=1004, "Noise"=1006] ("waveform")
                            n48 = call <instrlib>:"ww128x Configure Standard Waveform.vi"("amplitude"=w195, "frequency"=w193, "waveform"=w194, "instrument handle"=w192) -> ("error out"=w191:errorcluster)  [unwired: 4 in, 3 out]
                          }
                          frame 0 {
                            n49 = case shown="1, Default" w199 {
                              selector: w199 -> [w203 w205]
                              tunnel: [w203 w204] -> w198
                              frame 0 {
                              }
                              frame 1, Default {
                                n50 = expression code="(x+2)*5"(w205) -> (w204:i32)
                              }
                            }
                            n51 = Number To Decimal String(number=w198) -> (decimal integer string=w202:string)  [unwired: 1 in]
                            n52 = Concatenate Strings(":AMP " ("string"), w202) -> (w201:string)
                            n53 = call "Daxsonics Read Write.vi"("write buffer"=w201, "VISA resource name"=w197) -> ("error out"=w196:errorcluster)  [unwired: 7 in, 2 out]
                          }
                        }
                      }
                      frame #1 {
                        n54 = Wait (ms)(milliseconds to wait=500) -> ()  [unwired: 1 out]
                      }
                      frame #2 {
                        n55 = while {
                          tunnel: w221 -> [w243]
                          tunnel: [w242] -> w220
                          tunnel: [w241] -> w219
                          tunnel: [w240] -> w218
                          tunnel: [w239] -> w217
                          tunnel: w216 -> [w238]
                          tunnel: w215 -> [w237]
                          tunnel: w214 -> [w236]
                          tunnel: w213 -> [w231]
                          tunnel: w212 -> [w230]
                          tunnel: [w229] -> w211
                          tunnel: [w228] -> w210
                          tunnel: [w227] -> w209
                          tunnel: [w226] -> w208
                          tunnel: w207 -> [w222]
                          i -> [w235]
                          stop <- w224 stop-if-true
                          n56 = stacked-sequence {
                            seq-local: [w247 _ _] -> [_ w332 _]
                            seq-local: [w246 _ _] -> [_ _ w349]
                            tunnel: w243 -> [w264 w339 _]
                            tunnel: [w263 _ _] -> w242
                            tunnel: [w260 _ _] -> w241
                            tunnel: [w259 _ _] -> w240
                            tunnel: [w245 _ _] -> w239
                            tunnel: w238 -> [w258 _ _]
                            tunnel: w237 -> [_ w327 w350]
                            tunnel: w236 -> [_ w340 w360]
                            tunnel: [_ w326 _] -> w232
                            tunnel: w231 -> [w257 w335 _]
                            tunnel: w230 -> [w256 w325 w348]
                            tunnel: [w253 _ _] -> w229
                            tunnel: [w252 _ _] -> w228
                            tunnel: [w251 _ _] -> w227
                            tunnel: [_ w326 _] -> w225
                            tunnel: [w248 _ _] -> w226
                            tunnel: [_ _ w344] -> w223
                            tunnel: w222 -> [w244 _ _]
                            frame #0 {
                              # "Get data from CH0 (hydrophone)\nGet data from CH1 (Ref Voltage at Xducer)"
                              n57 = for {
                                N: "Average" -> [_]
                                tunnel: [w280] -> w265 mode=indexing
                                tunnel: w264 -> [w277]
                                tunnel: [w279] -> w262 mode=indexing
                                tunnel: [w278] -> w261 mode=indexing
                                tunnel: [w268] -> w245
                                tunnel: w258 -> [w276]
                                tunnel: w257 -> [w274]
                                tunnel: w256 -> [w273]
                                tunnel: [w271] -> w254 mode=indexing
                                tunnel: [w270] -> w255 mode=indexing
                                tunnel: [w269] -> w249 mode=indexing
                                tunnel: [w268] -> w247 mode=indexing
                                tunnel: [w267] -> w246 mode=indexing
                                tunnel: w244 -> [w266]
                                n58 = case shown="\"NI Digitizer\", Default" w274 {
                                tunnel: w277 -> [w289 _]
                                tunnel: w276 -> [w287 w301]
                                tunnel: [w286 w300] -> w268
                                tunnel: w273 -> [_ w318]
                                tunnel: [_ w309] -> w267
                                tunnel: w266 -> [w281 w296]
                                frame "Acqiris Digitizer" {
                                w288 = 1
                                n59 = call <instrlib>:"Configure Memory Settings.vi"("Number of Samples (1000)"=w287, "Number of Segments (1)"=w288, "Instrument ID"=w289) -> ("error out"=w282:errorcluster, "dup Instrument ID"=w285:u32)  [unwired: 1 in, 2 out]
                                n60 = call "conSamp.vi"("error in"=w282, "Digitizer Settings"=w281, "InstrumentID"=w285) -> ("error out"=w283:errorcluster, "DUP ID"=w284:u32)  [unwired: 1 in]
                                n61 = call <instrlib>:"Start Acquisition.vi"("error in (no error)"=w283, "Instrument ID"=w284) -> ("error out"=w293:errorcluster, "dup Instrument ID"=w294:u32)  [unwired: 2 in]
                                n62 = call <instrlib>:"Wait For End Of Acquisition.vi"("error in (no error)"=w293, "Timeout"=300, "Instrument ID"=w294) -> ("error out"=w291:errorcluster, "dup Instrument ID"=w292:u32)  [unwired: 3 out]
                                n63 = call "GetWaveform.vi"("Acq ID Out"=w292, "Read Mode"=enum32{"ADC", "Volts"}."Volts", "Num Samps"=w287, "Num Segs"=w288, "error in"=w291) -> ("first row"=w286:dbl[])  [unwired: 1 in, 9 out]
                                }
                                frame "NI Digitizer", Default {
                                n64 = property class="niScope"(reference=w318, "Min Number of Points"=w301, "Number of Records"=1) -> (reference out=w314:refnum<k15>, error out=w313:errorcluster)  [unwired: 1 in]
                                n65 = Bundle By Name(cluster=w296, "rf points per line"=1.0 ("Delay (micro s)")) -> ()  [unwired: 1 out]
                                n66 = call "NI conSamp.vi"("error in"=w313, "Digitizer Settings"=w296, "InstrumentID"=w314) -> ("error out"=w315:errorcluster, "DUP ID"=w316:refnum<k15>)  [unwired: 1 in]
                                n67 = call <instrlib>:"niScope Initiate Acquisition.vi"("instrument handle"=w316, "error in"=w315) -> ("instrument handle out"=w320:refnum<k15>, "error out"=w321:errorcluster)  [unwired: 12 out]
                                n68 = call-poly <instrlib>:"niScope Fetch (poly).vi"("timeout"=0.5, "error in"=w321, "numSamples"=w301, "channels"="0", "instrument handle"=w320) -> ("error out"=w303:errorcluster, "wfm"=w298:dbl[], "instrument handle out"=w305:refnum<k15>)  [unwired: 4 out]
                                n69 = call "NI conSamp.vi"("error in"=w303, "Digitizer Settings"=w296, "InstrumentID"=w305) -> ("error out"=w307:errorcluster, "DUP ID"=w308:refnum<k15>)  [unwired: 1 in]
                                n70 = call <instrlib>:"niScope Initiate Acquisition.vi"("instrument handle"=w308, "error in"=w307) -> ("instrument handle out"=w304:refnum<k15>, "error out"=w306:errorcluster)  [unwired: 12 out]
                                n71 = call-poly <instrlib>:"niScope Fetch (poly).vi"("timeout"=0.5, "error in"=w306, "numSamples"=w301, "channels"="1", "instrument handle"=w304) -> ("wfm"=w309:dbl[])  [unwired: 6 out]
                                n72 = Negate(x=w298) -> (-x=w299:dbl[])
                                n73 = Select(t=w299, s="Invert PAL voltage", f=w298) -> (s? t:f=w300:dbl[])
                                }
                                }
                                n74 = call-poly <vilib>:"Mean.vi"("X"=w267) -> ("mean"=w272:dbl)  [unwired: 1 out]
                                n75 = call-poly <vilib>:"Mean.vi"("X"=w268) -> ("mean"=w275:dbl)  [unwired: 1 out]
                                n76 = Subtract(x=w267, y=w272) -> ()  [unwired: 1 out]
                                n77 = Subtract(x=w268, y=w275) -> ()  [unwired: 1 out]
                                n78 = call-poly <vilib>:"RMS.vi"("X"=w268) -> ("rms value"=w271:dbl)  [unwired: 1 out]
                                n79 = call-poly <vilib>:"RMS.vi"("X"=w267) -> ("rms value"=w269:dbl)  [unwired: 1 out]
                                n80 = Array Max & Min(array=w268) -> (max value=w278:dbl, min value=w279:dbl)  [unwired: 2 out]
                                n81 = Array Max & Min(array=w267) -> (max value=w270:dbl)  [unwired: 3 out]
                                n82 = Subtract(x=w278, y=w279) -> (x-y=w280:dbl)
                              }
                              n83 = call-poly <vilib>:"Mean.vi"("X"=w261) -> ("mean"=w260:dbl)  [unwired: 1 out]
                              n84 = call-poly <vilib>:"Mean.vi"("X"=w254) -> ("mean"=w253:dbl)  [unwired: 1 out]
                              n85 = call-poly <vilib>:"Mean.vi"("X"=w255) -> ("mean"=w252:dbl)  [unwired: 1 out]
                              n86 = call-poly <vilib>:"Mean.vi"("X"=w265) -> ("mean"=w263:dbl)  [unwired: 1 out]
                              n87 = call-poly <vilib>:"Mean.vi"("X"=w249) -> ("mean"=w248:dbl)  [unwired: 1 out]
                              n88 = call-poly <vilib>:"Mean.vi"("X"=w262) -> ("mean"=w259:dbl)  [unwired: 1 out]
                              n89 = Divide(x=w248, y=w253) -> (x/y=w251:dbl)
                            }
                            frame #1 {
                              w323 = "0" ("Active Channel")
                              # "Check for +/- clipping and adapt voltage range on cH0"
                              n90 = Absolute Value(x=w332) -> (abs(x)=w331:dbl[][])
                              n91 = expression code="-X/2"(w327) -> (w328:dbl[])
                              n92 = Array Max & Min(array=w331) -> (max value=w330:dbl)  [unwired: 3 out]
                              n93 = Negate(x=w330) -> (-x=w329:dbl)
                              n94 = property class="niScope"(reference=w325, "Active Channel"=w323) -> (reference out=w322:refnum<k15>, "Vertical Range"=w324:dbl)  [unwired: 1 in, 1 out]
                              n95 = Multiply(x=w329, y=1.1) -> (x*y=w338:dbl)
                              n96 = Threshold 1D Array(2:w338, 3:w328) -> (0:w336:dbl)  [unwired: 1 out]
                              n97 = Round Toward -Infinity(1:w336) -> (0:w334:dbl)
                              n98 = Index Array(array=w327, index=w334) -> (element=w333:dbl)
                              n99 = Equal?(x=w333, y=w324) -> (x = y?=w326:bool)
                              n100 = case shown="True" w326 {
                                tunnel: w333 -> [w341 _]
                                tunnel: w340 -> [_ _]
                                tunnel: w339 -> [_ _]
                                tunnel: w335 -> [_ _]
                                tunnel: w323 -> [w343 _]
                                tunnel: w322 -> [w342 _]
                                frame False {
                                n101 = property class="niScope"(reference=w342, "Active Channel"=w343, "Vertical Range"=w341) -> ()  [unwired: 1 in, 2 out]
                                }
                                frame True {
                                }
                              }
                            }
                            frame #2 {
                              w344 = TRUE
                              (unwired) TRUE
                              w345 = "1" ("Active Channel")
                              # "Check for +/- clipping and adapt voltage range ON cH1"
                              n102 = Absolute Value(x=w349) -> (abs(x)=w354:dbl[][])
                              n103 = expression code="-X/2"(w350) -> (w351:dbl[])
                              n104 = Array Max & Min(array=w354) -> (max value=w353:dbl)  [unwired: 3 out]
                              n105 = property class="niScope"(reference=w348, "Active Channel"=w345) -> (reference out=w347:refnum<k15>, "Vertical Range"=w346:dbl)  [unwired: 1 in, 1 out]
                              n106 = Negate(x=w353) -> (-x=w352:dbl)
                              n107 = Multiply(x=w352, y=1.1) -> (x*y=w359:dbl)
                              n108 = Threshold 1D Array(2:w359, 3:w351) -> (0:w357:dbl)  [unwired: 1 out]
                              n109 = Round Toward -Infinity(1:w357) -> (0:w356:dbl)
                              n110 = Index Array(array=w350, index=w356) -> (element=w355:dbl)
                              n111 = Equal?(x=w355, y=w346) -> ()  [unwired: 1 out]
                              n112 = case shown="False" w344 {
                                tunnel: w347 -> [w363 _]
                                tunnel: w355 -> [w361 _]
                                tunnel: w360 -> [_ _]
                                tunnel: w345 -> [w362 _]
                                frame False {
                                n113 = property class="niScope"(reference=w363, "Active Channel"=w362, "Vertical Range"=w361) -> ()  [unwired: 1 in, 2 out]
                                }
                                frame True {
                                }
                              }
                            }
                          }
                          n114 = Equal?(x=10, y=w235) -> (x = y?=w233:bool)
                          n115 = Or(x=w232, y=w233) -> ()  [unwired: 1 out]
                          n116 = And(x=w223, y=w225) -> (x .and. y?=w224:bool)
                        }
                      }
                    }
                  }
                  n117 = Bundle(cluster=T11 {"+ pk Ch1"=[], "Pk-Pk Ch1"=[], "-Pk Ch1"=[], "V Steps"=[], "WaveForms Ch1"=[], "RMS Ch1"=[], "+  pk Ch2"=[], "RMS Ch2"=[], "RMS Ratio"=[], "freq"=0.0}, "+ pk Ch1"=w131, "Pk-Pk Ch1"=w118, "-Pk Ch1"=w130, "V Steps"=w125, "WaveForms Ch1"=w129, "RMS Ch1"=w117, "+  pk Ch2"=w116, "RMS Ch2"=w115, "RMS Ratio"=w112, "freq"=w114) -> (w127:T11)
                }
              }
            }
          }
          event "Save Cal Data": Value Change {
            n118 = event-data() -> ()  [unwired: 7 out]
            n119 = property on="Hydrophone" class="Enum (strict)"() -> ("RingText.Text"=w373:string)  [unwired: 2 in, 2 out]
            n120 = Concatenate Strings(w373, "\tFG drive (mVpp) \tvoltage at transducer (+Vp)\tvolt hydrop (-Vp)\tPressure Neg (MPa)\tvolt hydrop (+Vp)\tPressure Pos (MPa)", "\r\n") -> (w368:string)
            n121 = local read "Cal Array"() -> (w366:dbl[][])
            n122 = Array To Spreadsheet String(array=w366, 3:"%f" ("spreadsheet string")) -> (spreadsheet string=w369:string)  [unwired: 1 in]
            n123 = Concatenate Strings(w368, w369) -> (w367:string)
            n124 = Write to Text File(text=w367) -> ()  [unwired: 3 in, 3 out]
          }
          event "Save RF array?": Value Change {
            n125 = event-data() -> ()  [unwired: 7 out]
            n126 = local read "Raw RF"() -> (w378:dbl[][])
            n127 = call-poly <vilib>:"Write Delimited Spreadsheet.vi"("2D data"=w378, "transpose? (no:F)"=TRUE) -> ()  [unwired: 12 in, 2 out]
          }
          event "Set up Digi": Value Change {
            n128 = event-data() -> ()  [unwired: 2 out]
            n129 = call "SetUpDigi.vi"("Digitizer Settings"=w384, "Motion Settings In"=w383, "Type of scan"=ScanType2."M scan", "Therapy (T)"="Burst Select") -> ("Digitizer Settings Out"=w381:T1, "Motion Settings Out"=w382:T5)  [unwired: 9 in, 5 out]
          }
          event "V probe", "Freq Step to View": Value Change {
            n130 = event-data() -> ()  [unwired: 7 out]
            n131 = local read "Freq Steps"() -> (w397:u32)
            n132 = Decrement(x=w397) -> (x-1=w396:u32)
            n133 = Unbundle By Name("Pressure Cal Parameters") -> ("Hydrophone"=w418:T10, "booster amp?"=w387:bool)
            n134 = In Range and Coerce(upper limit=w396, x="Freq Step to View", lower limit=u8 0) -> (coerced(x)=w391:u32, In Range?=w395:bool)
            n135 = case shown="False" w395 {
              tunnel: w391 -> [w419 _]
              frame False {
                n136 = local write "Freq Step to View"(w419) -> ()
              }
              frame True {
              }
            }
            n137 = for {
              tunnel: w387 -> [w455]
              tunnel: w400 -> [w453] mode=indexing
              tunnel: w418 -> [w452]
              tunnel: [w451] -> w416 mode=concatenating
              tunnel: [w425] -> w415
              tunnel: [w437] -> w410 mode=concatenating
              tunnel: [w436] -> w408 mode=indexing
              tunnel: [w435] -> w406 mode=indexing
              tunnel: [w422] -> w404 mode=indexing
              tunnel: [w427] -> w394 mode=concatenating
              tunnel: [w424] -> w392 mode=indexing
              # "Intensity"
              # "FG drive\nvoltage matching (Vp)\nvolt hydrop -Vpk\nPressure  neg MPa"
              n138 = Unbundle By Name(w453) -> ("+ pk Ch1"=w421:dbl[], "Pk-Pk Ch1"=w444:dbl[], "-Pk Ch1"=w433:dbl[], "V Steps"=w425:dbl[], "WaveForms Ch1"=w450:dbl[][], "+  pk Ch2"=w426:dbl[], "freq"=w430:dbl, "RMS Ratio"=w423:dbl[])
              n139 = call "FindHydSens.vi"("booster amp?"=w455, "Frequency (MHz)"=w430, "Hydrophone"=w452) -> ("Sensitivity in Pa/V"=w454:dbl)  [unwired: 2 out]
              n140 = expression code="x*10**-6"(w454) -> (w443:dbl)
              "Mpa/V" <- w443
              n141 = Transpose 2D Array(2D array=w450) -> (transposed array=w445:dbl[][])
              n142 = Array Size(array=w425) -> (size(s)=w431:i32)
              n143 = Bundle("V Steps"=w425, "RMS Ratio"=w423) -> (w424:cluster{"V Steps":dbl[], "RMS Ratio":dbl[]})  [unwired: 1 in]
              n144 = Initialize Array(w430, w431) -> (w429:dbl[])
              n145 = Build Array(w421, w433) -> (w422:dbl[][])
              n146 = Build Array (concatenate)(w429, w425, w445) -> (w428:dbl[][])
              n147 = Transpose 2D Array(2D array=w428) -> (transposed array=w427:dbl[][])
              n148 = Multiply(x=w443, y=w421) -> (x*y=w420:dbl[])
              n149 = Multiply(x=w443, y=w444) -> (x*y=w442:dbl[])
              n150 = Multiply(x=w443, y=w433) -> (x*y=w434:dbl[])
              n151 = Absolute Value(x=w434) -> (abs(x)=w432:dbl[])
              n152 = Bundle("V Steps"=w425, w442) -> (w440:cluster{"V Steps":dbl[], dbl[]})  [unwired: 1 in]
              n153 = Bundle("V Steps"=w425, w420) -> (w439:cluster{"V Steps":dbl[], dbl[]})  [unwired: 1 in]
              n154 = Bundle("V Steps"=w425, w432) -> (w441:cluster{"V Steps":dbl[], dbl[]})  [unwired: 1 in]
              n155 = Build Array(w439, w440, w441) -> (w436:cluster{"V Steps":dbl[], dbl[]}[])
              n156 = Multiply(x=w426, y="V probe") -> (x*y=w456:dbl[])
              n157 = call <vilib>:"Linear Fit.vi"("Y"=w434, "X"=w425) -> ("slope"=→"slope":dbl, "intercept"=→"intercept":dbl, "residue"=→"mse":dbl)  [unwired: 4 in, 7 out]
              n158 = expression code="x*x*100/1.5"(w434) -> ()  [unwired: 1 out]
              n159 = Bundle("V Steps"=w425, w456) -> (w435:cluster{"V Steps":dbl[], dbl[]})  [unwired: 1 out]
              n160 = Initialize Array(w430, 3 ("dimension size")) -> (w437:dbl[])
              n161 = Build Array(w456, w433, w434, w421, w420) -> (w451:dbl[][])
            }
            n162 = Index Array(array=w400, index=w391) -> (element=w402:T11)
            n163 = Index Array(array=w392, index=w391) -> (element=→"RMS dB ratio":cluster{"V Steps":dbl[], "RMS Ratio":dbl[]})
            n164 = Unbundle By Name(w402) -> ("freq"=→"f (MHz)":dbl)
            n165 = Index Array(array=w404, index (dim 0)=w391) -> (element=→"Voltage + pk and -pk":dbl[][])  [unwired: 2 in]
            n166 = Transpose 2D Array(2D array=w394) -> (transposed array=→"Raw RF":dbl[][])
            n167 = Index Array(array=w408, index (row)=w391) -> (element=→"Hydrophone":cluster{"V Steps":dbl[], dbl[]}[])  [unwired: 1 in]
            n168 = Index Array(array=w406, index=w391) -> (element=→"Voltage at Transducer":cluster{"V Steps":dbl[], dbl[]})
            n169 = Build Array (concatenate)(0.0, w410) -> (w413:dbl[])
            n170 = Build Array (concatenate)(w415, w416) -> (w412:dbl[][])
            n171 = Transpose 2D Array(2D array=w412) -> (transposed array=w417:dbl[][])
            n172 = Build Array (concatenate)(w413, w417) -> (→"Cal Array":dbl[][])
          }
        }
      }
    }
    frame #2 {
      n173 = case shown="True" w457 {
        frame False {
        }
        frame True {
        }
      }
      n174 = case shown="7" w460 {
        tunnel: w459 -> [_ w462]
        tunnel: w458 -> [w461 _]
        frame 2, Default {
          n175 = call <instrlib>:"ag33xxx - Close.vi"("VISA session"=w461) -> ()  [unwired: 10 in, 1 out]
        }
        frame 7 {
          n176 = call <instrlib>:"ww128x Close.vi"("instrument handle"=w462) -> ()  [unwired: 1 in, 10 out]
        }
      }
    }
  }
  "Motion Settings Out" <- w2
  "Digitizer Settings Out" <- w1
  n177 = case shown="True" w6 {
    tunnel: w8 -> [_ w463]
    frame False {
    }
    frame True {
      n178 = call <instrlib>:"niScope Close.vi"("instrument handle"=w463) -> ()  [unwired: 1 in, 14 out]
    }
  }
